vi "Shooting.vi"(11 "Output Cluster in":T1) -> ()   [LabVIEW 2015]
uses:
  Joytsick/Controls to Cmmnds Output Clust.ctl
  Global Vars.vi
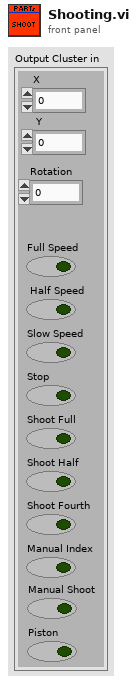
[diagram p1: front panel]
types:
  T1 = typedef "Controls to Cmmnds Output Clust.ctl" = cluster{"X ":dbl, " Y":dbl, "Rotation":dbl, "Full Speed":bool, " Half Speed":bool, "Slow Speed":bool, "Stop":bool, "Shoot Full":bool, "Shoot Half":bool, "Shoot Fourth":bool, "Manual Index":bool, "Piston":bool, "Manual Shoot":bool}
  T2 = typedef "WPI_MotorControlDeviceRef.ctl" = cluster{"DeviceStatus":errorcluster, "Type":T3, "PWM":cluster{"PWM Channel":T4, "DeadBand":T5}, "CAN":cluster{"Device Number":u8, "Control Mode":T6, "Semaphore":T7, "Max Vout":dbl, "TalonSRX Control Mode":T8}, "Invert":bool}
  T3 = typedef "WPI_MotorControlType.ctl" = enum16{"PWM", "CAN", "CANTalonSRX"}
  T4 = typedef "FPGA_DIOPWMChannel.ctl" = enum8{"PWM 0", "PWM 1", "PWM 2", "PWM 3", "PWM 4", "PWM 5", "PWM 6", "PWM 7", "PWM 8", "PWM 9", "PWM MXP 0", "PWM MXP 1", "PWM MXP 2", "PWM MXP 3", "PWM MXP 4", "PWM MXP 5", "PWM MXP 6", "PWM MXP 7", "PWM MXP 8", "PWM MXP 9", "Invalid"}
  T5 = typedef "WPI_PWMDeadband.ctl" = cluster{"Name":string, "maxPositivePwm":i32, "minPositivePwm":i32, "centerPwm":i32, "maxNegativePwm":i32, "minNegativePwm":i32, "angularRange":u16}
  T6 = typedef "WPI_CANJaguar_ControlMode.ctl" = enum8{"Percent VBus", "Current", "Speed", "Position", "Voltage"}
  T7 = typedef "Semaphore RefNum" = refnum<k1>
  T8 = typedef "WPI_CANTalonSRX_APIControlMode.ctl" = enum8{"Percent VBus", "Speed", "Position", "Slave", "Unchanged / Invalid", "Voltage Compensation", "Current", "Motion Profile"}
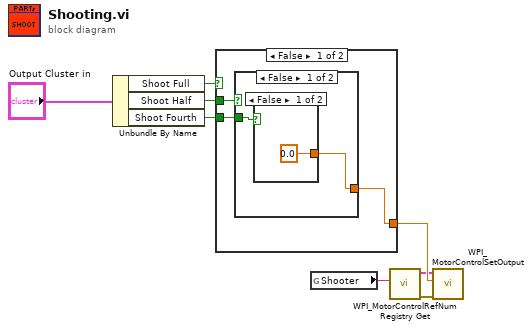
[diagram p0: block diagram]
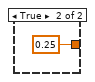
[diagram p2: hidden frame]
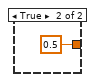
[diagram p3: hidden frame]
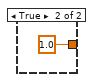
[diagram p4: hidden frame]
diagram:
  n1 = Unbundle By Name("Output Cluster in") -> ("Shoot Full"=w5:bool, "Shoot Half"=w7:bool, "Shoot Fourth"=w8:bool)
  n2 = case shown="False" w5 {
    tunnel: [w10 1.0] -> w6
    tunnel: w7 -> [w11 _]
    tunnel: w8 -> [w9 _]
    frame False {
      n3 = case shown="False" w11 {
        tunnel: [w13 0.5] -> w10
        tunnel: w9 -> [w12 _]
        frame False {
          n4 = case shown="False" w12 {
            tunnel: [0.0 0.25] -> w13
            frame False {
            }
            frame True {
            }
          }
        }
        frame True {
        }
      }
    }
    frame True {
    }
  }
  n5 = global read "Global Vars.vi" "Shooter"() -> (w2:string)
  n6 = call <vilib>:"WPI_MotorControlRefNum Registry Get.vi"("refnum name"=w2) -> ("error out"=w4:errorcluster, "MotorControlDevRef"=w3:T2)  [unwired: 9 in]
  n7 = call <vilib>:"WPI_MotorControlSetOutput.vi"("error in (no error)"=w4, "Output"=w6, "MotorControlDevRef"=w3) -> ()  [unwired: 6 in, 3 out]
